vi "Get Then Set VISA Timeout.vi"(0 "VISA Resource Name In":refnum<visa-resource-name>, 5 "New Timeout (msecs)":u32=3000, 11 "error in (no error)":errorcluster, 12 "Max Timeout (300 secs)":u32=300000, 13 "Min Timeout (3 secs)":u32=3000) -> (4 "VISA Resource Name Out (dupl)":refnum<visa-resource-name>, 6 "Old Timeout (msecs)":u32=3000, 8 "Actual Set Timeout (msecs)":u32=3000, 15 "error out":errorcluster)   [LabVIEW 2010, in "Keithley 622x.lvlib"]
doc: "Both returns the current VISA timeout and sets a new timeout. This is useful in VIs that need to temporarily change the VISA timeout at the start of the VI, then reset it back to the original value when the VI completes."
uses:
  Keithley 622x.lvlib
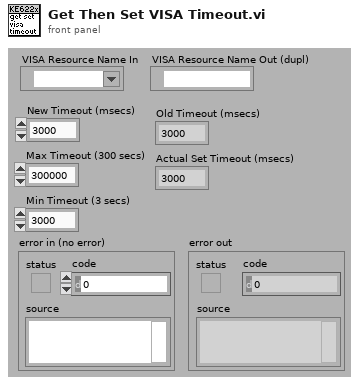
[diagram p1: front panel]
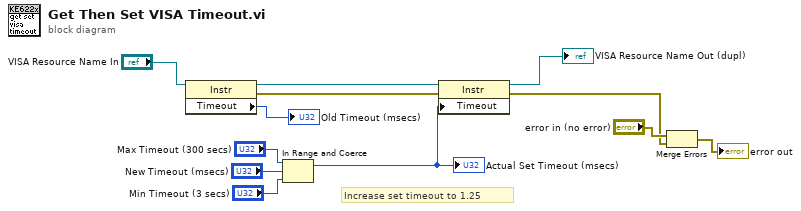
[diagram p0: block diagram]
diagram:
  # "Increase set timeout to 1.25"
  n1 = property class="Instr"(reference="VISA Resource Name In") -> (reference out=w10:refnum<visa-resource-name>, error out=w11:errorcluster, "Timeout"=→"Old Timeout (msecs)":u32)  [unwired: 1 in]
  n2 = In Range and Coerce(upper limit="Max Timeout (300 secs)", x="New Timeout (msecs)", lower limit="Min Timeout (3 secs)") -> (coerced(x)=w5:u32)  [unwired: 1 out]
  "Actual Set Timeout (msecs)" <- w5
  n3 = property class="Instr"(reference=w10, error in=w11, "Timeout"=w5) -> (reference out=→"VISA Resource Name Out (dupl)":refnum<visa-resource-name>, error out=w3:errorcluster)
  n4 = Merge Errors("error in (no error)", w3) -> (→"error out":errorcluster)
